vi "Configure Calc Compare Pass.vi"(6 "Calculate Compare PASS LO (0: Off)":u16(ring) format="%_1g" items=["Off", "On"], 7 "Calculate Compare PASS HI (0: Off)":u16(ring) format="%_1g" items=["Off", "On"], 8 "error in (no error)":errorcluster, 10 "Calculate Compare PASS GO (1: On)":u16(ring)=1 format="%_1g" items=["Off", "On"], 11 "VISA resource name":refnum<visa-resource-name>) -> (0 "error out":errorcluster, 3 "VISA resource name out":refnum<visa-resource-name>)   [LabVIEW 2017, in "ADCMT7451_ADC.lvlib"]
doc: "This VI configures PASS condition."
uses:
  ADCMT7451_ADC.lvlib
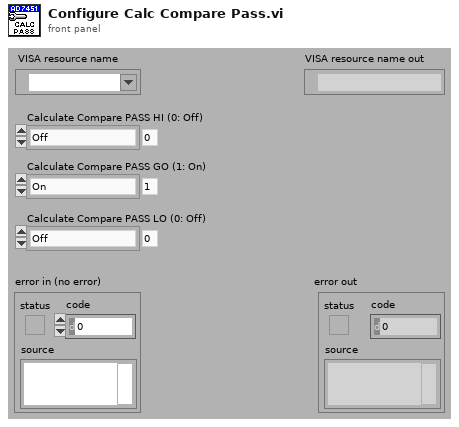
[diagram p1: front panel]
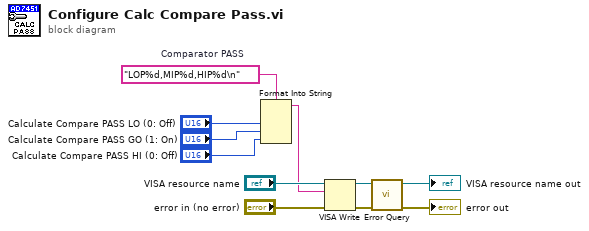
[diagram p0: block diagram]
diagram:
  w5 = "LOP%d,MIP%d,HIP%d\n"  # Comparator PASS
  n1 = Format Into String(format string=w5, "Calculate Compare PASS LO (0: Off)", "Calculate Compare PASS GO (1: On)", "Calculate Compare PASS HI (0: Off)") -> (resulting string=w1:string)  [unwired: 2 in, 1 out]
  n2 = VISA Write(VISA resource name="VISA resource name", write buffer=w1, error in (no error)="error in (no error)") -> (VISA resource name out=w7:refnum<visa-resource-name>, error out=w6:errorcluster)  [unwired: 1 out]
  n3 = call "Error Query.vi"("error in (no error)"=w6, "VISA resource name"=w7) -> ("error out"=→"error out":errorcluster, "VISA resource name out"=→"VISA resource name out":refnum<visa-resource-name>)  [unwired: 6 in, 2 out]
